vi "OAT Orbit Probe Angle Compensation.vi"(2 "probe angle compensation":u16(ring) items=["0", "45", "90", "135", "180", "225", "270", "315"], 3 "XY plot data in":cluster{dbl[], dbl[]}[](array[cluster]) {"?" format="%.2f"; "?" format="%.2f"}) -> (1 "XY plot data out":cluster{dbl[], dbl[]}[](array[cluster]) {"?" format="%.2f"; "?" format="%.2f"})   [LabVIEW 2017]
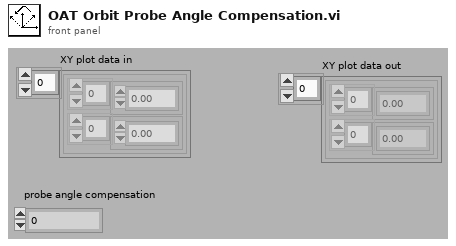
[diagram p1: front panel]
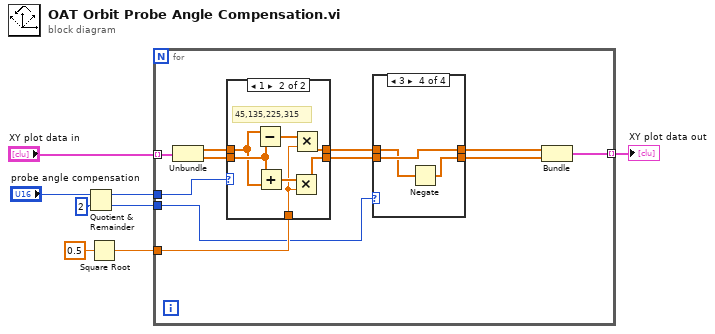
[diagram p0: block diagram]
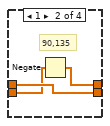
[diagram p3: hidden frame]
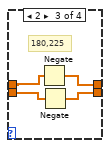
[diagram p4: hidden frame]
diagram:
  n1 = Quotient & Remainder(x="probe angle compensation", y=u16 2) -> (x-y*floor(x/y)=w5:u16, floor(x/y)=w2:u16)
  n2 = Square Root(x=0.5) -> (sqrt(x)=w3:dbl)
  n3 = for {
    tunnel: "XY plot data in" -> [w16] mode=indexing
    tunnel: [w17] -> w7 mode=indexing
    tunnel: w5 -> [w15]
    tunnel: w3 -> [w14]
    tunnel: w2 -> [w13]
    n4 = Unbundle(w16) -> (w19:dbl[], w18:dbl[])
    n5 = case shown="1" w15 {
      tunnel: w18 -> [w32 w40]
      tunnel: w19 -> [w33 w39]
      tunnel: [w33 w35] -> w12
      tunnel: [w32 w34] -> w10
      tunnel: w14 -> [_ w36]
      frame 0, Default {
        # "0,90,180,270"
      }
      frame 1 {
        # "45,135,225,315"
        n6 = Subtract(x=w39, y=w40) -> (x-y=w38:dbl[])
        n7 = Add(x=w40, y=w39) -> (x+y=w37:dbl[])
        n8 = Multiply(x=w37, y=w36) -> (x*y=w34:dbl[])
        n9 = Multiply(x=w38, y=w36) -> (x*y=w35:dbl[])
      }
    }
    n10 = case shown="3" w13 {
      tunnel: w12 -> [w21 w24 w28 w30]
      tunnel: [w21 w22 w27 w31] -> w11
      tunnel: w10 -> [w20 w23 w26 w31]
      tunnel: [w20 w24 w25 w29] -> w9
      frame 0, Default {
        # "0,45"
      }
      frame 1 {
        # "90,135"
        n11 = Negate(x=w23) -> (-x=w22:dbl[])
      }
      frame 2 {
        # "180,225"
        n12 = Negate(x=w28) -> (-x=w27:dbl[])
        n13 = Negate(x=w26) -> (-x=w25:dbl[])
      }
      frame 3 {
        n14 = Negate(x=w30) -> (-x=w29:dbl[])
      }
    }
    n15 = Bundle(w11, w9) -> (w17:cluster{dbl[], dbl[]})  [unwired: 1 in]
  }
  "XY plot data out" <- w7
